vi "Writer.vi"() -> ()   [LabVIEW 2020]
panel:
  in  "Cluster":T1
  in  "OK Button":bool
  out "concatenated string":string
  in  "stop":bool
  out "error out":errorcluster
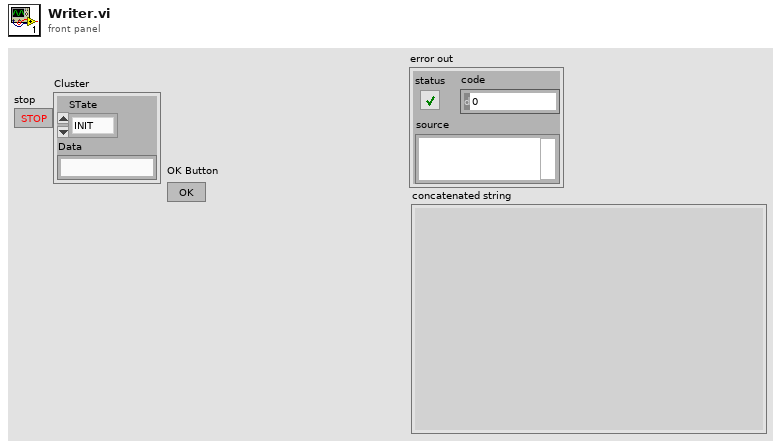
[diagram p1: front panel]
types:
  T1 = cluster{"STate":enum16{"INIT", "EROR", "MESG", "STOP"}, "Data":string}
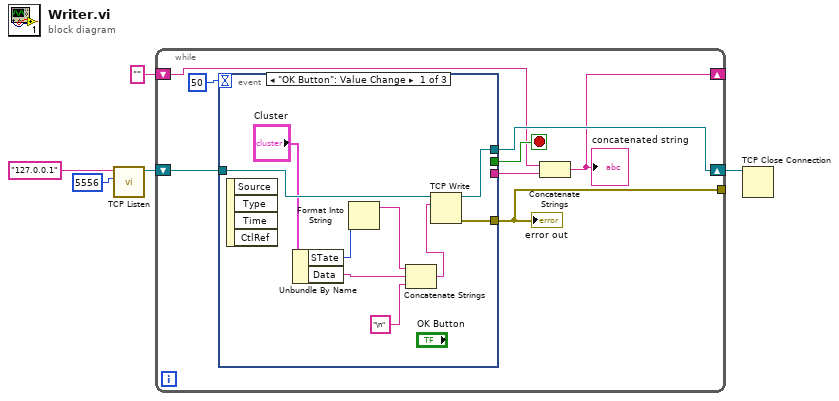
[diagram p0: block diagram]
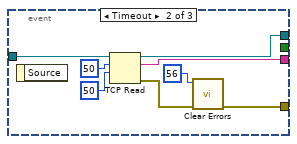
[diagram p2: hidden frame]
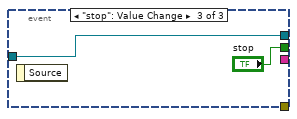
[diagram p3: hidden frame]
diagram:
  n1 = call <vilib>:"TCP Listen.vi"("port"=u16 5556, "service name"="127.0.0.1") -> ("connection ID"=w3:refnum<k5>)  [unwired: 5 in, 4 out]
  n2 = while {
    tunnel: [w12] -> _
    shift-right: [w10] -> w2
    shift-left: w3 -> [w13]
    shift-right: [w8] -> _
    shift-left: "" -> [w7]
    stop <- w11 stop-if-true
    n3 = event shown="[0] \"OK Button\": Value Change" {
      selector: _ -> [_ _ _]
      dyn-events: _ -> [_ _ _]
      timeout: 50 -> [_ _ _]
      tunnel: w13 -> [w22 w30 w31]
      tunnel: [w21 w28 _] -> w12
      tunnel: [_ _ "stop"] -> w11
      tunnel: [w20 w25 w31] -> w10
      tunnel: [_ w24 _] -> w9
      event "OK Button": Value Change {
        n4 = event-data() -> ()  [unwired: 1 in, 4 out]
        n5 = Unbundle By Name("Cluster") -> ("STate"=w17:enum16{"INIT", "EROR", "MESG", "STOP"}, "Data"=w14:string)
        n6 = Format Into String(w17) -> (resulting string=w15:string)  [unwired: 3 in, 1 out]
        n7 = Concatenate Strings(w15, w14, "\n" ("string")) -> (w19:string)
        n8 = TCP Write(connection ID=w22, data in=w19) -> (connection ID out=w20:refnum<k5>, error out=w21:errorcluster)  [unwired: 2 in, 1 out]
      }
      event Timeout {
        n9 = event-data() -> ()  [unwired: 1 in, 1 out]
        n10 = TCP Read(connection ID=w30, bytes to read=50, 9:50 ("timeout ms (25000)")) -> (connection ID out=w25:refnum<k5>, data out=w24:string, error out=w26:errorcluster)  [unwired: 2 in]
        n11 = call <vilib>:"Clear Errors.vi"("error in (no error)"=w26, "specific error code to clear (0: all)"=56) -> ("error out"=w28:errorcluster)  [unwired: 4 in, 1 out]
      }
      event "stop": Value Change {
        n12 = event-data() -> ()  [unwired: 1 in, 1 out]
      }
    }
    "error out" <- w12
    n13 = Concatenate Strings(w7, w9) -> (w8:string)
    "concatenated string" <- w8
  }
  n14 = TCP Close Connection(connection ID=w2) -> ()  [unwired: 2 in, 2 out]
